vi "PH_GUI.set waveform graph II GUI object.vi"(2 "WaveformGraph in":refnum<vi>, 3 "Array":waveform(dbl)[](array[waveform]), 5 "error in (no error)":errorcluster) -> (19 "error out":errorcluster)   [LabVIEW 2014, in "PH_Common.lvlib"]
uses:
  PH_Common.lvlib
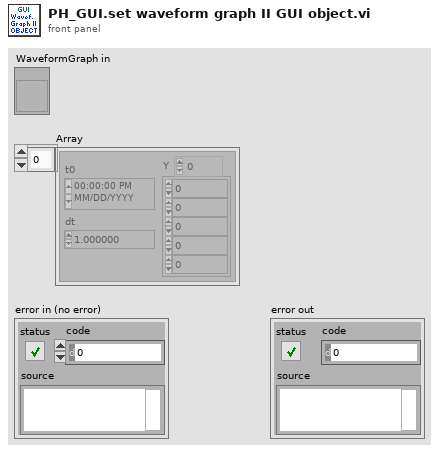
[diagram p1: front panel]
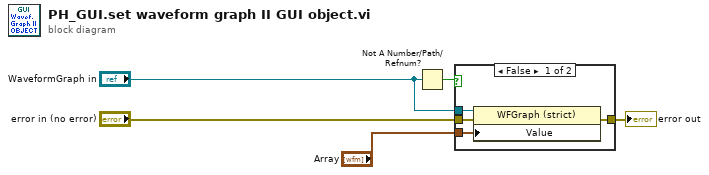
[diagram p0: block diagram]
diagram:
  n1 = Not A Number/Path/Refnum?(number/path/refnum="WaveformGraph in") -> (NaN/Path/Refnum?=w4:bool)
  n2 = case shown="False" w4 {
    tunnel: "Array" -> [w9 _]
    tunnel: "error in (no error)" -> [w8 w10]
    tunnel: [w7 w10] -> w3
    tunnel: "WaveformGraph in" -> [w6 _]
    frame False {
      n3 = property class="WFGraph (strict)"(reference=w6, error in=w8, "Value"=w9) -> (error out=w7:errorcluster)  [unwired: 1 out]
    }
    frame True {
    }
  }
  "error out" <- w3
